vi "Dashboard Main.vi"() -> ()   [LabVIEW 2016]
uses:
  <vilib>/event_ctls.llb/eventvkey.ctl
  <vilib>/Rock Robotics/WPI/Dashboard/WPI_DashboardLogging Global.vi
  <vilib>/Utility/miscctls.llb/LVRowAndColumnTypeDef.ctl
  <vilib>/Rock Robotics/Network Tables/NT Write Boolean.vi
  <vilib>/Rock Robotics/Network Tables/NT Read Numeric Array.vi
panel:
  out "error out":errorcluster
  out "error out 2":errorcluster
  in  "Camera Settings Right":T1={"Frame Rate"=30, "Compression"=30, "Size"=1, "DB Camera Config"=FALSE} {"Frame Rate" scale=1.0..30.0; "Compression" scale=100.0..-1.0; "Size" items=["640x480", "320x240", "160x120"]}
  in  "Camera Name Right":string(combo)="No Camera Selection"
  out "Camera Info":cluster{"Mbps LED":bool, "Mbps":dbl, "fps":dbl} {"fps" format="%#.1g"; "Mbps" format="%#.1g"}
  in  "Camera Settings":T1={"Frame Rate"=30, "Compression"=30, "Size"=1, "DB Camera Config"=FALSE} {"Frame Rate" scale=1.0..30.0; "Compression" scale=100.0..-1.0; "Size" items=["640x480", "320x240", "160x120"]}
  in  "TCP":refnum<k5>
  in  "Rec Mode":enum32{"Stop", "Record", "Playback"}(radio)
  out "Robot IP":string
  out "Image Message":string="Timeout in Camera Communications"
  in  "Dashboard Tab":T2(tab)
  in  "Select Auto":string(combo)="Select Autonomous ..."
  out "NT Connection":bool
  out "MotorChart R":cluster{"Numeric":dbl, "Numeric":dbl}(graph)
  out "MotorChart L":cluster{"Numeric":dbl, "Numeric":dbl}(graph)
  out "MotorSliders R":cluster{"MotorSlide1":dbl, "MotorSlide2":dbl} {"MotorSlide2" scale=-1.0..1.0 scale format="%#_2e"; "MotorSlide1" scale=-1.0..1.0 scale format="%#_2e"}
  out "MotorSliders L":cluster{"MotorSlide1":dbl, "MotorSlide2":dbl} {"MotorSlide2" scale=-1.0..1.0 scale format="%#_2e"; "MotorSlide1" scale=-1.0..1.0 scale format="%#_2e"}
  out "JS1 Z":dbl(slide) scale=-1.0..1.0 scale format="%#_2e"
  out "JS1 Graph":cluster{"X":dbl, "Y":dbl}[](graph)
  out "JS1 Buttons":T3
  out "JS2 Z":dbl(slide) scale=-1.0..1.0 scale format="%#_2e"
  out "JS2 Graph":cluster{"X":dbl, "Y":dbl}[](graph)
  out "JS2 Buttons":T3
  out "Mode":T4(ring)=enum."Auto Disabled"
  out "Gear State":string="Waiting...."
  in  "Mode 2":bool
  out "Camera Image Right":T5(plugin-control)
  in  "DB/String 9":string
  in  "DB/String 8":string
  in  "DB/String 7":string
  in  "DB/String 6":string
  in  "DB/String 5":string
  in  "DB/String 4":string
  in  "DB/String 3":string
  in  "DB/String 2":string
  in  "DB/String 1":string
  in  "DB/String 0":string
  in  "DB/Slider 0":dbl(slide) scale=0.0..5.0
  in  "DB/Slider 1":dbl(slide) scale=0.0..5.0
  in  "DB/Slider 2":dbl(slide) scale=0.0..5.0
  in  "DB/Slider 3":dbl(slide) scale=0.0..5.0
  out "DB/LED 3":bool
  out "DB/LED 2":bool
  out "DB/LED 1":bool
  out "DB/LED 0":bool
  in  "DB/Button 3":bool
  in  "DB/Button 2":bool
  in  "DB/Button 1":bool
  in  "DB/Button 0":bool caption="New Name"
  in  "Test Slider":dbl(slide) scale=0.0..100.0 scale format="%#_3g"
  in  "On/Off":bool caption="Solenoid"
  in  "Test Name":u16(ring) items=["Select the test to run..."]
  in  "Test Tree":string(tree)
  in  "Motor":cluster{"Value":dbl, "Enable":bool} {"Value" scale=-1.0..1.0 scale format="%#_3g"}
  out "Progress":T6 {"Test Progress" scale=0.0..100.0}
  in  "Rev/Fwd":cluster{"Forward":bool, "Reverse":bool}
  in  "Test Ring":u16(ring) items=["Monochrome", "Color"]
  out "Cmd Status":string
  in  "Execute Command":bool
  in  "Command Params":string[][](table)
  in  "Command Selection":i32(listbox)
  in  "CheckList":i32(listbox)
  out "Tree":string(tree)
  in  "Max Speed":dbl=1.0 format="%#_13g"
  in  "Foreward Sensitivity":dbl=1.0 format="%#_13g"
  in  "Turning Sensitivity":dbl=0.4 format="%#_13g"
  in  "High Gear Turning Multiplier":dbl=0.65 format="%#_13g"
  in  "High Gear":bool=TRUE
  in  "Direction Toggle":bool=TRUE
  in  "Autoshift":bool=TRUE
  in  "Save":bool
  in  "Load":bool
  in  "Profile Name":string="Profile1"
  out "Camera Image":T5(plugin-control)
  out "Background":bool
  in  "Camera Name":string(combo)="No Camera Selection"
  # "HW"
  # "HW"
  # "Joysticks"
  # "Drive Motors"
  # "Front"
  # "Right"
  # "Left"
  # "Back"
  # "This tab is a great place for autonomous settings and robot-specific values.\nPlace controls and indicators inside this tab and match name to\nDashboard Variables on robot. You can also delete this comment."
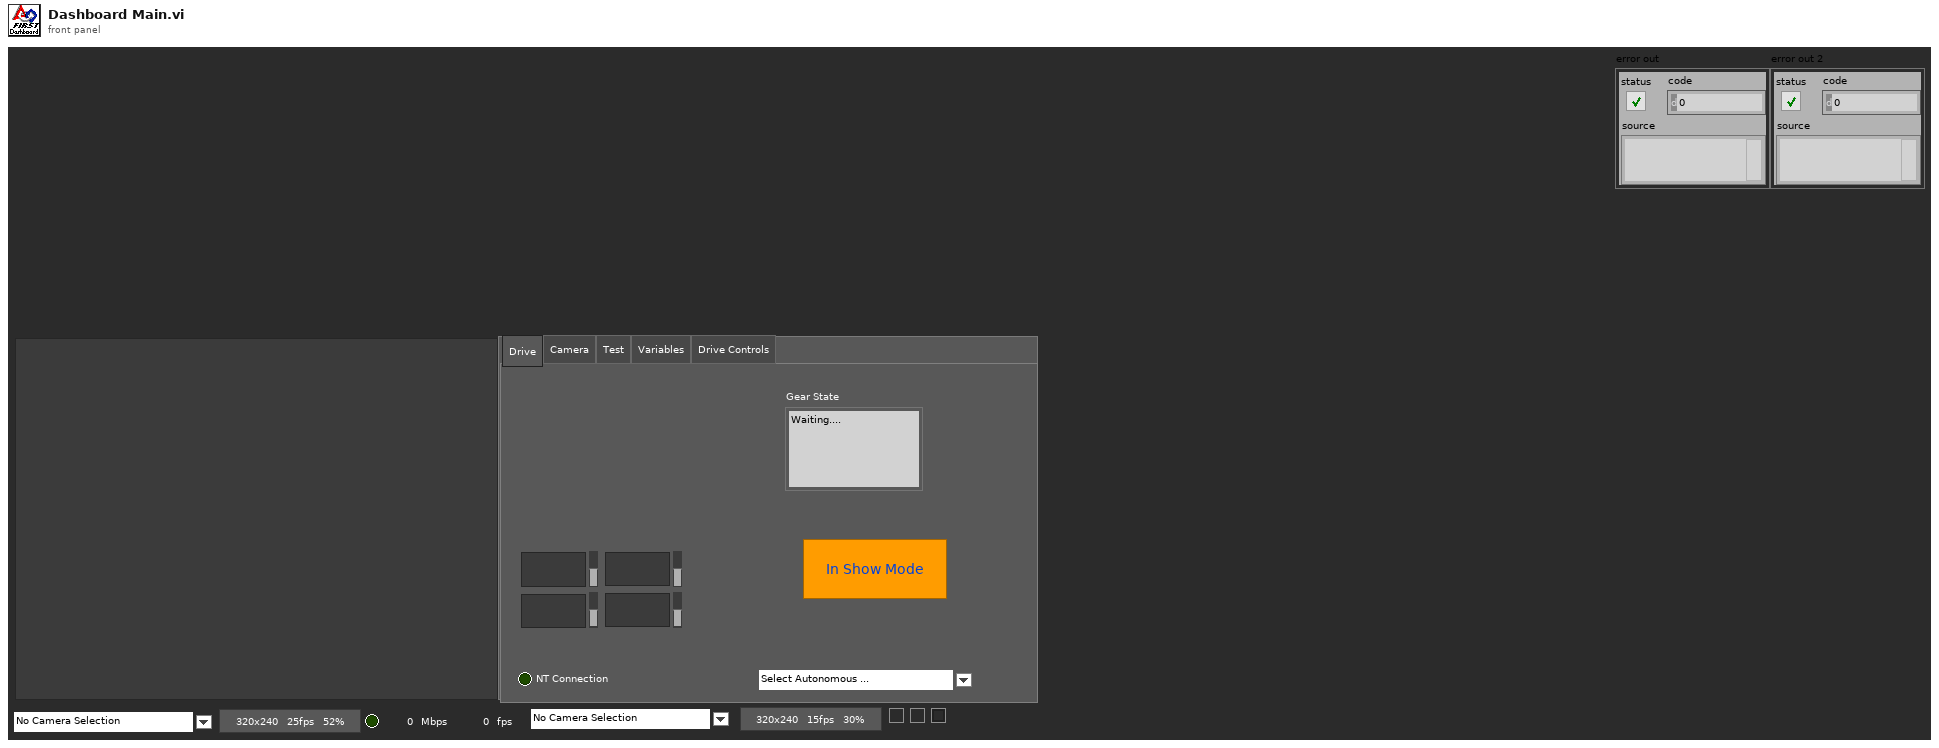
[diagram p1: front panel]
types:
  T1 = cluster{"Frame Rate":i32, "Compression":i32, "Size":u16, "DB Camera Config":bool}
  T2 = enum32{"Drive", "Camera", "Basic", "Custom", "Test", "Commands", "Checklist", "Variables", "Drive Controls"}
  T3 = cluster{bool, bool, bool, bool, bool, bool, bool, bool, bool, bool, bool, bool}
  T4 = enum8{"Tele-Op Disabled", "Tele-Op Enabled", "Auto Disabled", "Auto Enabled", "Test Disabled", "Test Enabled", "Disconnected", "No Code", "E-Stop"}
  T5 = typedef "IMAQ Image.ctl" = refnum<image>
  T6 = cluster{"Test Progress":u8, "Test Progress Text":string}
  T7 = typedef "Image Type" = u32
  T8 = cluster{"IDs":cluster{"RPC field ID":u16, "Unique ID":u16}, "String":string}
  T9 = enum32{"Drive", "Camera", "Basic", "Custom", "Test", "Commands", "Checklist", "Variables"}
  T10 = enum32{"Drive", "Basic", "Custom", "Test", "Checklist", "Variables"}
  T11 = cluster{"Error Strings":string, "Disable Counts":cluster{u16, u16}, "Rail Faults":cluster{u16, u16, u16}, "Robot IP":string, "DB Mode":u8, "Event Info":cluster{"Name":string, "Type":u8, "Number":u16, "Replay":u8}}
  T12 = cluster{"Storage":cluster{"Disk Free":u64, "RAM Block":u32, "RAM free":u32}, "CPU Utilization":cluster{"CPU % ISR":sgl, "CPU % Time Crit":sgl, "CPU % Timed Str":sgl, "CPU % High":sgl, "CPU % Above":sgl, "CPU % Normal":sgl, "CPU % Low":sgl}, "CAN":cluster{"% Bus Utilization":sgl, "Bus Off Cnt":u32, "TX_FIFO Full Cnt":u32, "Receive Error Cnt":u8, "Transmit Error Cnt":u8}, "HID":cluster{"HID Outputs":u32, "Rumble Low":u16, "Rumble High":u16}[]}
  T13 = cluster{"Status bits":cluster{"Test Mode":bool, "Autonomous":bool, "Enabled":bool, "Code Start":bool, "Brownout":bool, "Reserved 2":bool, "Reserved 3":bool, "E-Stop":bool}, "Code Trace":cluster{"Disabled":bool, "TeleOp":bool, "Auto":bool, "Test":bool}, "Controller Type":enum16{"unknown", "cRIO", "roboRio"}, "Code?":enum16{"unknown", "noCode", "code"}, "Battery V":dbl}
  T14 = cluster{"Control Bits":cluster{"TestMode":bool, "Autonomous":bool, "Enabled":bool, "FMS Present":bool, bool, bool, bool, "E-Stop":bool}, "Team Station ":u8, "Countdown":sgl, "Joystick Values":cluster{"Axes":dbl[], "Buttons":bool[], "POVs":i16[]}[]}
  T15 = cluster{"Axes":dbl[], "Buttons":bool[], "POVs":i16[]}[]
  T16 = cluster{"Axes":dbl[], "Buttons":bool[], "POVs":i16[]}
  T17 = cluster{"Buttons[0]":bool, "Buttons[1]":bool, "Buttons[2]":bool, "Buttons[3]":bool, "Buttons[4]":bool, "Buttons[5]":bool, "Buttons[6]":bool, "Buttons[7]":bool, "Buttons[8]":bool, "Buttons[9]":bool, "Buttons[10]":bool, "Buttons[11]":bool}
  T18 = cluster{"Camera Image":refnum<vi>, "Dashboard Tab":refnum<vi>, "Background":refnum<vi>, "Rec Mode":refnum<vi>, "Test Slider":refnum<vi>, "On/Off ":refnum<vi>, "Test Ring":refnum<vi>, "Rev/Fwd":refnum<vi>, "Test Name":refnum<vi>, "Motor":refnum<vi>, "Progress":refnum<vi>, "CheckList":refnum<vi>, "Tree":refnum<vi>, "Test Tree":refnum<vi>, "Command Params":refnum<vi>, "Command Selection":refnum<vi>, "Execute Command":refnum<vi>, "Cmd Status":refnum<vi>, "Camera Settings":refnum<vi>, "Camera Name":refnum<vi>, "Camera Info":refnum<vi>, "Camera Settings Right":refnum<vi>, "Camera Name Right":refnum<vi>, "Camera Image Right":refnum<vi>}
  T19 = cluster{"Operation":enum16{"Update", "Clear"}, "Color Box":u32}[]
  T20 = typedef "eventvkey.ctl" = enum16{"ASCII", "Enter", "Return", "Shift", "Ctrl", "Alt", "Cmd", "Opt", "Caps", "NumLock", "Clear", "Break", "Up", "Down", "Left", "Right", "Insert", "Delete", "Home", "End", "PageUp", "PageDown", "Escape", "Help", "Pause", "ScrollLock", "F1", "F2", "F3", "F4", "F5", "F6", "F7", "F8", "F9", "F10", "F11", "F12", "F13", "F14", "F15", "F16", "F17", "F18", "F19", "F20", "F21", "F22", "F23", "F24", "Play", "VolumeUp", "VolumeDown", "Mute", "Two Byte Char"}
  T21 = cluster{"Image Size":bool, "Image Type":bool, "Pixel Value":bool, "ROI Information":bool, "Zoom Factor":bool}
  T22 = cluster{"Operation":enum16{"Update", "Clear"}, "Color Box":u32}
  T23 = typedef "LVRowAndColumnTypeDef.ctl" = cluster{"Row":i32, "Column":i32}
  T24 = cluster{"Shift":bool, "Ctrl":bool, "Alt":bool, "Cmd":bool, "Opt":bool}
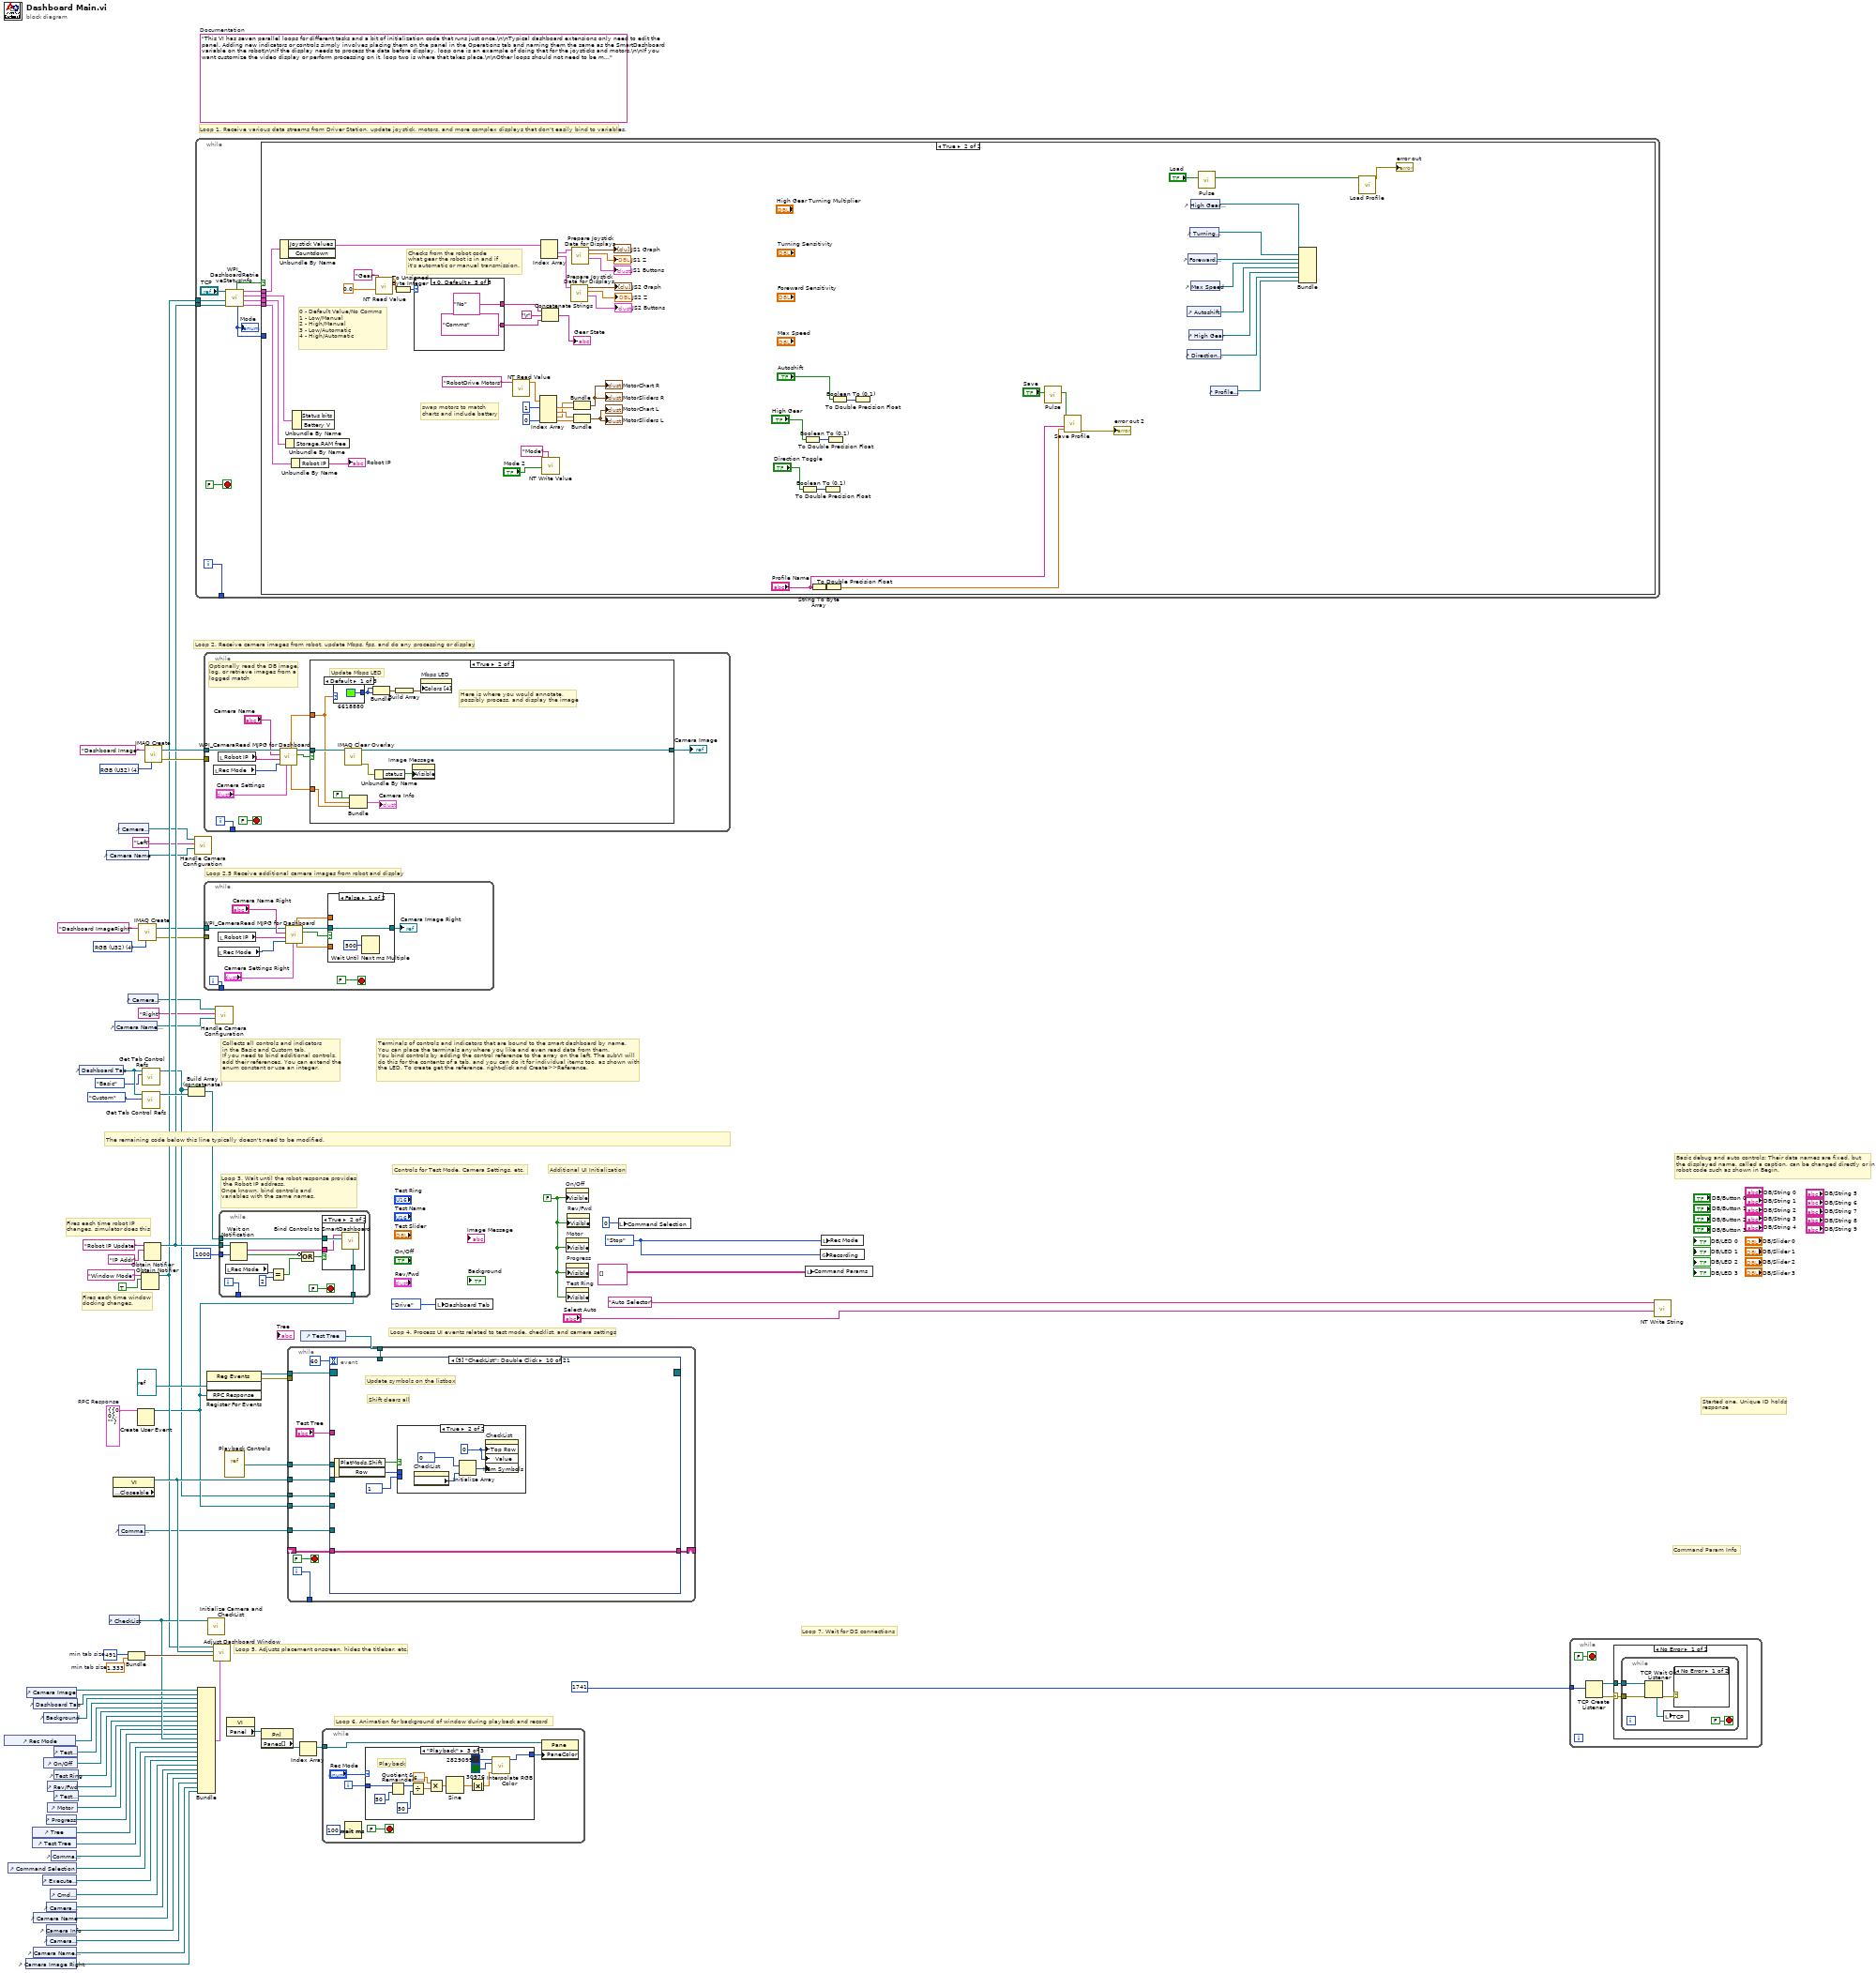
[diagram p0: block diagram]
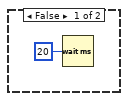
[diagram p3: hidden frame]
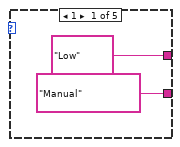
[diagram p4: hidden frame]
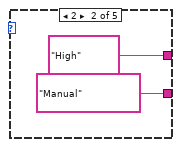
[diagram p5: hidden frame]
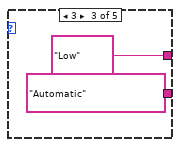
[diagram p6: hidden frame]
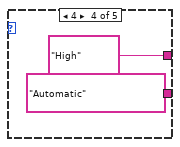
[diagram p7: hidden frame]
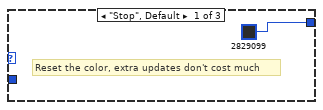
[diagram p8: hidden frame]
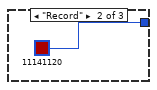
[diagram p9: hidden frame]
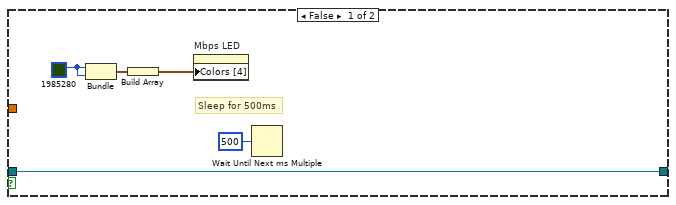
[diagram p11: hidden frame]
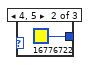
[diagram p12: hidden frame]
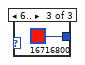
[diagram p13: hidden frame]
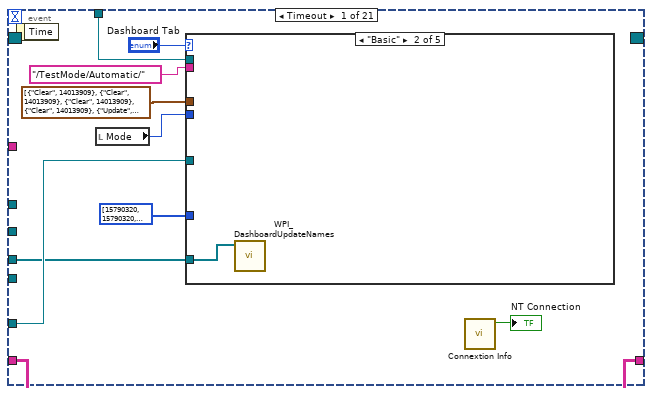
[diagram p14: hidden frame]
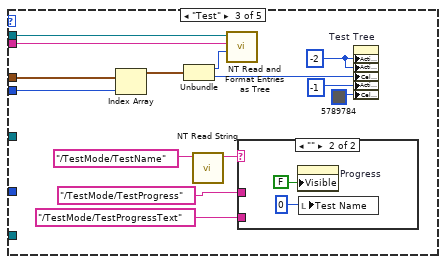
[diagram p16: hidden frame]
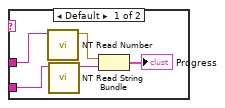
[diagram p17: hidden frame]
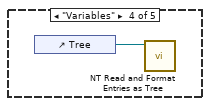
[diagram p18: hidden frame]
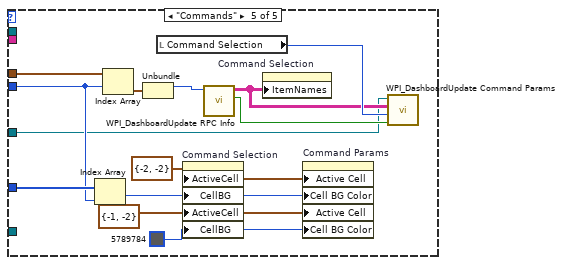
[diagram p19: hidden frame]
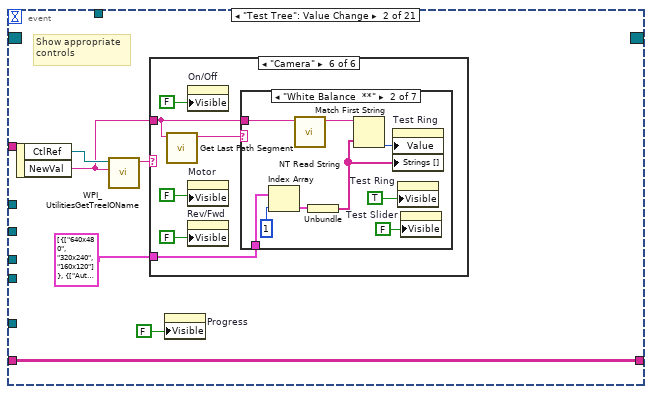
[diagram p20: hidden frame]
diagram:
  w10 = T7 4 items=["Grayscale (U8)", "Grayscale (I16)", "Grayscale (SGL)", "Complex (CSG)", "RGB (U32)", "HSL (U32)", "RGB (U64)"] ("Image Type")
  w26 = T8 {"IDs"={"RPC field ID"=0, "Unique ID"=0}, "String"=""}  # RPC Response
  w51 = 491  # min tab size
  w50 = 1.333  # min tab size
  w58 = enum32{"Stop", "Record", "Playback"}."Stop" ("Rec Mode")
  w33 = FALSE ("Visible")
  (unwired) "This VI has seven parallel loops for different tasks and a bit of initialization code that runs just once.\n\nTypical dashboard extensions only need to edit the panel. Adding new indicators or controls simply involves placing them on the panel in the Operations tab and naming them the same as the SmartDashboard variable on the robot\n\nIf the display needs to process the data before display, loop one is an example of doing that for the joysticks and motors.\n\nIf you want customize the video display or perform processing on it, loop two is where that takes place.\n\nOther loops should not need to be modified. They are pretty standard, and document the task they perform."  # Documentation
  w75 = T7 4 items=["Grayscale (U8)", "Grayscale (I16)", "Grayscale (SGL)", "Complex (CSG)", "RGB (U32)", "HSL (U32)", "RGB (U64)"] ("Image Type")
  # "Loop 2.5 Receive additional camera images from robot and display"
  # "Command Param Info"
  # "Started one, Unique ID holds\nresponse"
  # "Loop 7. Wait for DS connections"
  # "Basic debug and auto controls: Their data names are fixed, but\nthe displayed name, called a caption, can be changed directly or in\nrobot code such as shown in Begin."
  # "Controls for Test Mode, Camera Settings, etc."
  # "Additional UI Initialization"
  # "Loop 6. Animation for background of window during playback and record"
  # "Fires each time robot IP\nchanges, simulator does this"
  # "Fires each time window\ndocking changes."
  # "Collects all controls and indicators\nin the Basic and Custom tab.\nIf you need to bind additional controls,\nadd their references. You can extend the\nenum constant or use an integer."
  # "The remaining code below this line typically doesn't need to be modified."
  # "Loop 4. Process UI events related to test mode, checklist, and camera settings"
  # "Terminals of controls and indicators that are bound to the smart dashboard by name.\nYou can place the terminals anywhere you like and even read data from them.\nYou bind controls by adding the control reference to the array on the left. The subVI will\ndo this for the contents of a tab, and you can do it for individual items too, as shown with\nthe LED. To create get the reference, right-click and Create>>Reference."
  # "Loop 3. Wait until the robot response provides\n the Robot IP address.\nOnce known, bind controls and\nvariables with the same names."
  # "Loop 5. Adjusts placement onscreen, hides the titlebar, etc."
  # "Loop 1. Receive various data streams from Driver Station, update joystick, motors, and more complex displays that don't easily bind to variables."
  # "Loop 2. Receive camera images from robot, update Mbps, fps, and do any processing or display"
  n1 = control-ref of="Rec Mode"() -> (w39:refnum<vi>)
  n2 = control-ref of="Command Selection"() -> (w25:refnum<vi>)
  n3 = control-ref of="Camera Image Right"() -> (w1:refnum<vi>)
  n4 = control-ref of="Camera Image"() -> (w53:refnum<vi>)
  n5 = control-ref of="Tree"() -> (w43:refnum<vi>)
  n6 = control-ref of="Test Tree"() -> (w42:refnum<vi>)
  n7 = control-ref of="Dashboard Tab"() -> (w52:refnum<vi>)
  n8 = control-ref of="Camera Name"() -> (w16:refnum<vi>)
  n9 = control-ref of="Camera Name Right"() -> (w2:refnum<vi>)
  n10 = control-ref of="Execute Command"() -> (w27:refnum<vi>)
  n11 = control-ref of="Background"() -> (w48:refnum<vi>)
  n12 = control-ref of="On/Off"() -> (w37:refnum<vi>)
  n13 = control-ref of="Progress"() -> (w34:refnum<vi>)
  n14 = control-ref of="Camera Settings"() -> (w17:refnum<vi>)
  n15 = control-ref of="Camera Info"() -> (w15:refnum<vi>)
  n16 = control-ref of="Camera Settings Right"() -> (w3:refnum<vi>)
  n17 = control-ref of="Rev/Fwd"() -> (w35:refnum<vi>)
  n18 = control-ref of="Motor"() -> (w40:refnum<vi>)
  n19 = control-ref of="Cmd Status"() -> (w21:refnum<vi>)
  n20 = control-ref of="Command Params"() -> (w28:refnum<vi>)
  n21 = control-ref of="Test Slider"() -> (w38:refnum<vi>)
  n22 = control-ref of="Test Ring"() -> (w36:refnum<vi>)
  n23 = control-ref of="Test Name"() -> (w41:refnum<vi>)
  n24 = control-ref of="Dashboard Tab"() -> (w56:refnum<vi>)
  n25 = control-ref of="Camera Name"() -> (w18:refnum<vi>)
  n26 = control-ref of="CheckList"() -> (w44:refnum<vi>)
  n27 = property class="VI" props=["Front Panel.Closeable"]() -> (reference out=w57:refnum<vi>)  [unwired: 2 in, 2 out]
  n28 = control-ref of="Camera Name Right"() -> (w6:refnum<vi>)
  n29 = control-ref of="Camera Settings"() -> (w19:refnum<vi>)
  n30 = control-ref of="Command Params"() -> (w20:refnum<vi>)
  n31 = control-ref of="Camera Settings Right"() -> (w7:refnum<vi>)
  n32 = Bundle("min tab size"=w51, "min tab size"=w50) -> (w49:cluster{"min tab size":i32, "min tab size":dbl})  [unwired: 1 in]
  n33 = Create User Event(user event datatype=w26) -> (user event=w22:refnum<user-event>)  [unwired: 1 in, 1 out]
  n34 = call "IMAQ Create"("Image Name"="Dashboard ImageRight", "Image Type"=w10) -> ("New Image"=w9:T5, "error out"=w8:errorcluster)  [unwired: 2 in, 1 out]
  n35 = Obtain Notifier(name (unnamed)="Window Mode", notification data type=TRUE) -> (notifier out=w31:refnum<notifier>)  [unwired: 2 in, 2 out]
  n36 = call <vilib>:"Get Tab Control Refs.vi"("Page Index"=T10."Basic" ("Dashboard Tab"), "TabControl in"=w56) -> ("ControlsOnPage"=w14:refnum<vi>[])  [unwired: 9 in]
  n37 = call <vilib>:"Get Tab Control Refs.vi"("Page Index"=T10."Custom" ("Dashboard Tab"), "TabControl in"=w56) -> ("ControlsOnPage"=w55:refnum<vi>[])  [unwired: 9 in]
  n38 = Obtain Notifier(name (unnamed)="Robot IP Update", notification data type="IP Addr" ("name (unnamed)")) -> (notifier out=w32:refnum<notifier>)  [unwired: 2 in, 2 out]
  n39 = call "IMAQ Create"("Image Name"="Dashboard Image", "Image Type"=w75) -> ("New Image"=w73:T5, "error out"=w72:errorcluster)  [unwired: 2 in, 1 out]
  n40 = Build Array (concatenate)(w14, w55) -> (w54:refnum<vi>[])
  n41 = call "Handle Camera Configuration.vi"("CameraNameRef"=w18, "Camera File Name"="Left", "ClusterRef"=w19) -> ()  [unwired: 9 in]
  n42 = while {
    tunnel: [w85] -> _
    tunnel: w32 -> [w79]
    tunnel: w31 -> [w76]
    i -> [w85]
    stop <- FALSE stop-if-true
    n43 = call <vilib>:"WPI_DashboardRetrieveStatusInfo.vi"("Binding Refnum"=w79, "Window Mode Notifier"=w76, "TCP Cnx"="TCP") -> ("Power and Errors"=w80:T11, "Robot Metrics"=w83:T12, "Status Info"=w84:T13, "Control Info"=w81:T14, "Robot Mode"=w78:T4, "Process?"=w82:bool)  [unwired: 3 in]
    "Mode" <- w78
    n44 = case shown="True" w82 {
      tunnel: w84 -> [_ w144]
      tunnel: w83 -> [_ w143]
      tunnel: w81 -> [_ w142]
      tunnel: w80 -> [_ w141]
      tunnel: w78 -> [_ _]
      frame False {
        n45 = Wait (ms)(milliseconds to wait=u32 20) -> ()  [unwired: 1 out]
      }
      frame True {
        # "Checks from the robot code\nwhat gear the robot is in and if\nit's automatic or manual transmission."
        # "0 - Default Value/No Comms\n1 - Low/Manual\n2 - High/Manual\n3 - Low/Automatic\n4 - High/Automatic"
        # "swap motors to match\ncharts and include battery"
        n46 = Unbundle By Name(w142) -> ("Joystick Values"=w132:T15)  [unwired: 1 out]
        n47 = Unbundle By Name(w143) -> ()  [unwired: 1 out]
        n48 = Unbundle By Name(w141) -> ("Robot IP"=→"Robot IP":string)
        n49 = Unbundle By Name(w144) -> ()  [unwired: 2 out]
        n50 = call-poly <vilib>:"NT Read Value.vi"("Default Value"=0.0, "Name"="Gear") -> ("Numeric"=w113:dbl)  [unwired: 8 in, 1 out]
        n51 = To Unsigned Byte Integer(number=w113) -> (unsigned 8bit integer=w114:u8)
        n52 = case shown="0, Default" w114 {
          tunnel: ["Low" "High" "Low" "High" "No"] -> w118
          tunnel: ["Manual" "Manual" "Automatic" "Automatic" "Comms"] -> w116
          frame 1 {
          }
          frame 2 {
          }
          frame 3 {
          }
          frame 4 {
          }
          frame 0, Default {
          }
        }
        n53 = call-poly <vilib>:"NT Read Value.vi"("Name"="RobotDrive Motors") -> ("Numeric Array"=w122:dbl[])  [unwired: 9 in, 1 out]
        n54 = Index Array(array=w122, index #1=1, index #4=0) -> (element #1=w136:dbl, element #2=w137:dbl, element #3=w135:dbl, element #4=w140:dbl)  [unwired: 2 in]
        n55 = Index Array(array=w132) -> (element #1=w131:T16, element #2=w127:T16)  [unwired: 2 in]
        n56 = Concatenate Strings(w118, "\r", w116) -> (→"Gear State":string)
        n57 = call-poly <vilib>:"NT Write Value.vi"("Boolean"="Mode 2", "Name"="Mode") -> ()  [unwired: 9 in, 1 out]
        n58 = call "Prepare Joystick Data for Displays.vi"("Joystick Values"=w127) -> ("Buttons"=→"JS2 Buttons":T17, "Z Axis"=→"JS2 Z":dbl, "Cartesian Data"=→"JS2 Graph":cluster{"X axis":dbl, "X axis":dbl}[])  [unwired: 8 in]
        n59 = call "Prepare Joystick Data for Displays.vi"("Joystick Values"=w131) -> ("Buttons"=→"JS1 Buttons":T17, "Z Axis"=→"JS1 Z":dbl, "Cartesian Data"=→"JS1 Graph":cluster{"X axis":dbl, "X axis":dbl}[])  [unwired: 8 in]
        n60 = Bundle("Numeric"=w135, "Numeric"=w136) -> (→"MotorChart R" →"MotorSliders R":cluster{"Numeric":dbl, "Numeric":dbl})  [unwired: 1 in]
        n61 = Bundle("Numeric"=w137, "Numeric"=w140) -> (→"MotorChart L" →"MotorSliders L":cluster{"Numeric":dbl, "Numeric":dbl})  [unwired: 1 in]
        n62 = Boolean To (0,1)(Boolean="Direction Toggle") -> (0, 1=w103:i16)
        n63 = Boolean To (0,1)(Boolean="High Gear") -> (0, 1=w102:i16)
        n64 = String To Byte Array(string="Profile Name") -> (unsigned byte array=w105:u8[])
        n65 = To Double Precision Float(number=w103) -> ()  [unwired: 1 out]
        n66 = To Double Precision Float(number=w105) -> (double precision float=w106:dbl[])
        n67 = To Double Precision Float(number=w102) -> ()  [unwired: 1 out]
        n68 = Boolean To (0,1)(Boolean="Autoshift") -> (0, 1=w101:i16)
        n69 = To Double Precision Float(number=w101) -> ()  [unwired: 1 out]
        n70 = call "Pulse.vi"("Input"="Save") -> ("Output"=w100:bool)  [unwired: 10 in]
        n71 = call "Save Profile.vi"("Array 2"=w106, "Profile Name"="Profile Name", "Output"=w100) -> ("error out"=→"error out 2":errorcluster)  [unwired: 8 in]
        n72 = control-ref of="Direction Toggle"() -> (w89:refnum<vi>)
        n73 = control-ref of="Autoshift"() -> (w91:refnum<vi>)
        n74 = control-ref of="Foreward Sensitivity"() -> (w93:refnum<vi>)
        n75 = control-ref of="High Gear"() -> (w90:refnum<vi>)
        n76 = control-ref of="Turning Sensitivity"() -> (w94:refnum<vi>)
        n77 = control-ref of="High Gear Turning Multiplier"() -> (w95:refnum<vi>)
        n78 = control-ref of="Max Speed"() -> (w92:refnum<vi>)
        n79 = call "Pulse.vi"("Input"="Load") -> ("Output"=w97:bool)  [unwired: 10 in]
        n80 = control-ref of="Profile Name"() -> (w88:refnum<vi>)
        n81 = Bundle("High Gear Turning Multiplier"=w95, "Turning Sensitivity"=w94, "Foreward Sensitivity"=w93, "Max Speed"=w92, "Autoshift"=w91, "High Gear"=w90, "Direction Toggle"=w89, "Profile Name"=w88) -> ()  [unwired: 1 in, 1 out]
        n82 = call "Load Profile.vi"("Output"=w97) -> ("error out"=→"error out":errorcluster)  [unwired: 14 in]
      }
    }
  }
  n83 = Bundle("Camera Image"=w53, "Dashboard Tab"=w52, "Background"=w48, "Rec Mode"=w39, "Test Slider"=w38, "On/Off"=w37, "Test Ring"=w36, "Rev/Fwd"=w35, "Test Name"=w41, "Motor"=w40, "Progress"=w34, "CheckList"=w44, "Tree"=w43, "Test Tree"=w42, "Command Params"=w28, "Command Selection"=w25, "Execute Command"=w27, "Cmd Status"=w21, "Camera Settings"=w17, "Camera Name"=w16, "Camera Info"=w15, "Camera Settings Right"=w3, "Camera Name Right"=w2, "Camera Image Right"=w1) -> (w45:T18)  [unwired: 1 in]
  n84 = while {
    tunnel: w73 -> [w164]
    tunnel: w72 -> [_]
    tunnel: [w165] -> _
    i -> [w165]
    stop <- FALSE stop-if-true
    # "Optionally read the DB image,\nlog, or retrieve images from a\nlogged match"
    n85 = local read "Rec Mode"() -> (w160:enum32{"Stop", "Record", "Playback"})
    n86 = local read "Robot IP"() -> (w159:string)
    n87 = call <vilib>:"WPI_CameraRead MJPG for Dashboard.vi"("Camera Settings"="Camera Settings", "Rec Mode"=w160, "Robot IP"=w159, "Camera Name"="Camera Name", "Refnum in"=w164) -> ("Active"=w162:bool, "Refnum out"=w163:T5, "FPS"=w161:dbl, "Bandwidth (Mbps)"=w158:dbl)  [unwired: 3 in]
    n88 = case shown="True" w162 {
      tunnel: w163 -> [w167 w178]
      tunnel: w158 -> [_ w175]
      tunnel: w161 -> [_ w176]
      tunnel: [w167 w172] -> w155
      frame False {
        w169 = u32 1985280 ("Color Box")
        # "Sleep for 500ms"
        n89 = Bundle("Color Box"=w169, "Color Box"=w169) -> (w170:cluster{"Color Box":u32, "Color Box":u32})  [unwired: 1 out]
        n90 = Build Array(w170) -> (w168:cluster{"Color Box":u32, "Color Box":u32}[])
        n91 = property on="Mbps LED" class="Bool (strict)"("Colors [4]"=w168) -> ()  [unwired: 2 in, 2 out]
        n92 = Wait Until Next ms Multiple(millisecond multiple=u32 500) -> ()  [unwired: 1 out]
      }
      frame True {
        # "Here is where you would annotate,\npossibly process, and display the image"
        # "Update Mbps LED"
        n93 = case shown="Default" w175 {
          tunnel: [u32 6618880 ("Color Box") u32 16776722 ("Color Box") u32 16716800 ("Color Box")] -> w179
          frame Default {
          }
          frame 4, 5 {
          }
          frame 6.. {
          }
        }
        n94 = call "IMAQ Clear Overlay"("Image"=w178) -> ("error out"=w181:errorcluster, "Image Out"=w172:T5)  [unwired: 2 in, 7 out]
        n95 = Bundle(FALSE, "Bandwidth (Mbps)"=w175, "FPS"=w176) -> (→"Camera Info":cluster{bool, "Bandwidth (Mbps)":dbl, "FPS":dbl})  [unwired: 1 in]
        n96 = Bundle("Color Box"=w179, "Color Box"=w179) -> (w180:cluster{"Color Box":u32, "Color Box":u32})  [unwired: 1 out]
        n97 = Unbundle By Name(w181) -> ("status"=w182:bool)
        n98 = Build Array(w180) -> (w177:cluster{"Color Box":u32, "Color Box":u32}[])
        n99 = property on="Image Message" class="Str"("Visible"=w182) -> ()  [unwired: 2 in, 2 out]
        n100 = property on="Mbps LED" class="Bool (strict)"("Colors [4]"=w177) -> ()  [unwired: 2 in, 2 out]
      }
    }
    "Camera Image" <- w155
  }
  n101 = while {
    tunnel: w9 -> [w196]
    tunnel: w8 -> [_]
    tunnel: [w190] -> _
    i -> [w190]
    stop <- FALSE stop-if-true
    n102 = local read "Rec Mode"() -> (w194:enum32{"Stop", "Record", "Playback"})
    n103 = local read "Robot IP"() -> (w195:string)
    n104 = call <vilib>:"WPI_CameraRead MJPG for Dashboard.vi"("Camera Settings"="Camera Settings Right", "Rec Mode"=w194, "Robot IP"=w195, "Camera Name"="Camera Name Right", "Refnum in"=w196) -> ("Active"=w189:bool, "Refnum out"=w192:T5, "FPS"=w187:dbl, "Bandwidth (Mbps)"=w188:dbl)  [unwired: 3 in]
    n105 = case shown="False" w189 {
      tunnel: w192 -> [w198 w200]
      tunnel: w188 -> [_ _]
      tunnel: w187 -> [_ _]
      tunnel: [w198 w200] -> w186
      frame False {
        n106 = Wait Until Next ms Multiple(millisecond multiple=u32 500) -> ()  [unwired: 1 out]
      }
      frame True {
      }
    }
    "Camera Image Right" <- w186
  }
  n107 = register-events(refnum<vi> refnum, w22) -> (reference out=w62:refnum<event-registration>, error out=w61:errorcluster)  [unwired: 2 in]
  n108 = call "Initialize Camera and CheckList.vi"("ListBox in"=w44) -> ()  [unwired: 11 in]
  n109 = call "Adjust Dashboard Window.vi"("Sizing Refnums"=w45, "Size Constraints"=w49, "VI"=w57, "WIn Mode"=w31) -> ()  [unwired: 8 in]
  n110 = call "Handle Camera Configuration.vi"("CameraNameRef"=w6, "Camera File Name"="Right", "ClusterRef"=w7) -> ()  [unwired: 9 in]
  n111 = while {
    tunnel: w54 -> [w212]
    tunnel: w32 -> [w210]
    tunnel: [w208] -> _
    tunnel: u32 1000 ("milliseconds to wait") -> [w207]
    tunnel: w22 -> [w201]
    i -> [w208]
    stop <- FALSE stop-if-true
    n112 = local read "Rec Mode"() -> (w203:enum32{"Stop", "Record", "Playback"})
    n113 = Wait on Notification(notifier=w210, timeout in ms (-1)=w207) -> (notification=w209:string, timed out?=w205:bool)  [unwired: 2 in, 2 out]
    n114 = Equal?(x=w203, y=u16 2 ("Rec Mode")) -> (x = y?=w204:bool)
    n115 = Compound Arithmetic op=OR(invert w205, w204) -> (w206:bool)
    n116 = case shown="True" w206 {
      tunnel: w212 -> [_ w215]
      tunnel: w209 -> [_ w214]
      tunnel: w201 -> [_ w213]
      frame False {
      }
      frame True {
        n117 = call <vilib>:"Bind Controls to SmartDashboard.vi"("RPC ref"=w213, "Bound Control Refs"=w215, "Server IP Address"=w214) -> ()  [unwired: 9 in]
      }
    }
  }
  n118 = vi-ref "Playback Controls.vi"() -> (w63:refnum<vi>)
  n119 = property class="VI"() -> ("Panel"=w65:refnum<vi>)  [unwired: 2 in, 2 out]
  n120 = property class="Pnl"(reference=w65) -> ("Panes[]"=w66:refnum<vi>[])  [unwired: 1 in, 2 out]
  n121 = Index Array(array=w66) -> (element=w64:refnum<vi>)  [unwired: 1 in]
  n122 = control-ref of="Test Tree"() -> (w67:refnum<vi>)
  n123 = while {
    tunnel: [w225] -> _
    tunnel: w67 -> [w224]
    tunnel: w63 -> [w223]
    tunnel: w62 -> [w222]
    tunnel: w61 -> [_]
    tunnel: w57 -> [w221]
    tunnel: w22 -> [w220]
    tunnel: w20 -> [w219]
    shift-right: [w218] -> _
    shift-left: _ -> [w217]
    tunnel: w14 -> [w216]
    i -> [w225]
    stop <- FALSE stop-if-true
    n124 = event shown="[9] \"CheckList\": Double Click" {
      selector: w222 -> [_ _ _ _ _ _ _ _ _ _ _ _ _ _ _ _ _ _ _ _ _]
      dyn-events: [_ _ _ _ _ _ _ _ _ _ _ _ _ _ _ _ w481 _ _ _ _] -> _
      timeout: u32 60 ("milliseconds to wait") -> [_ _ _ _ _ _ _ _ _ _ _ _ _ _ _ _ _ _ _ _ _]
      tunnel: w224 -> [w237 _ _ _ _ _ _ _ _ _ _ _ _ _ _ _ _ _ _ _ _]
      tunnel: "Test Tree" -> [_ _ _ _ _ _ _ _ _ _ _ w448 w456 w458 w462 w470 _ _ _ _ _]
      tunnel: w223 -> [_ _ _ _ _ _ _ _ _ _ _ _ _ _ _ _ w483 _ w501 _ _]
      tunnel: w221 -> [_ _ _ _ _ _ _ _ _ _ _ _ _ _ _ _ w479 _ _ _ _]
      tunnel: w220 -> [_ _ _ _ _ _ _ _ _ _ _ _ _ _ _ _ w475 _ _ _ _]
      tunnel: w219 -> [w232 _ _ _ _ _ w399 _ _ _ _ _ _ _ _ _ _ _ _ _ _]
      tunnel: [w231 w276 w378 w383 w392 w396 w397 w406 w416 w423 w435 w447 w454 w457 w461 w469 w474 w496 w498 w502 w513] -> w218
      tunnel: w217 -> [w231 w276 w378 w383 w392 w396 w397 _ _ w423 w435 w447 w454 w457 w461 w469 w474 w496 w498 w502 w513]
      tunnel: w216 -> [w229 _ _ _ _ _ _ _ _ _ _ _ _ _ _ _ _ _ _ _ _]
      event Timeout {
        n125 = event-data() -> ()  [unwired: 1 in, 1 out]
        n126 = local read "Mode"() -> (w234:T4)
        n127 = case shown="\"Basic\"" "Dashboard Tab" {
          tunnel: w237 -> [_ _ w253 _ _]
          tunnel: "/TestMode/Automatic/" ("Name Pattern") -> [_ _ w252 _ _]
          tunnel: T19 [{"Operation"=enum."Clear", "Color Box"=14013909}, {"Operation"=enum."Clear", "Color Box"=14013909}, {"Operation"=enum."Clear", "Color Box"=14013909}, {"Operation"=enum."Clear", "Color Box"=14013909}, {"Operation"=enum."Update", "Color Box"=14013909}, {"Operation"=enum."Update", "Color Box"=16777215}, {"Operation"=enum."Clear", "Color Box"=14013909}, {"Operation"=enum."Clear", "Color Box"=14013909}, {"Operation"=enum."Clear", "Color Box"=14013909}] -> [_ _ w245 _ w269]
          tunnel: w234 -> [_ _ w244 _ w268]
          tunnel: u32[] [15790320, 15790320, 15790320, 15790320, 16777215, 16777215, 15790320, 15790320, 15790320] -> [_ _ _ _ w274]
          tunnel: w232 -> [_ _ _ _ w262]
          tunnel: w229 -> [_ w239 _ _ _]
          frame "Custom", Default {
          }
          frame "Basic" {
            n128 = call <vilib>:"WPI_DashboardUpdateNames.vi"("Controls on Tab"=w239) -> ()  [unwired: 11 in]
          }
          frame "Test" {
            w251 = -2 ("Active Item:Row Number")
            n129 = Index Array(array=w245, index=w244) -> (element=w246:T22)
            n130 = Unbundle(w246) -> ("Operation"=w247:enum16{"Update", "Clear"}, "Color Box"=w248:u32)
            n131 = call <vilib>:"NT Read String.vi"("Name"="/TestMode/TestName") -> ("String"=w242:string)  [unwired: 9 in, 1 out]
            n132 = call <vilib>:"NT Read and Format Entries as Tree.vi"("Operation"=w247, "Name Pattern"=w252, "Tree Refnum"=w253) -> ()  [unwired: 7 in, 2 out]
            n133 = case shown="\"\"" w242 {
              tunnel: "/TestMode/TestProgress" ("Name") -> [w255 _]
              tunnel: "/TestMode/TestProgressText" ("Name") -> [w254 _]
              frame Default {
                n134 = call <vilib>:"NT Read Number.vi"("Name"=w255) -> ("Numeric"=w256:dbl)  [unwired: 9 in, 1 out]
                n135 = call <vilib>:"NT Read String.vi"("Name"=w254) -> ("String"=w257:string)  [unwired: 9 in, 1 out]
                n136 = Bundle("Numeric"=w256, "String"=w257) -> (→"Progress":cluster{"Numeric":dbl, "String":string})  [unwired: 1 in]
              }
              frame "" {
                n137 = property on="Progress" class="Clust (strict)"("Visible"=FALSE) -> ()  [unwired: 2 in, 2 out]
                n138 = local write "Test Name"(u16 0) -> ()
              }
            }
            n139 = property on="Test Tree" class="Tree (strict)"("Active Item Row Number"=w251, "ActiveColNum"=w251, "CellBG"=w248, "Active Item Row Number"=-1 ("Active Item:Row Number"), "CellBG"=u32 5789784 ("Color Box")) -> ()  [unwired: 2 in, 2 out]
          }
          frame "Variables" {
            n140 = control-ref of="Tree"() -> (w261:refnum<vi>)
            n141 = call <vilib>:"NT Read and Format Entries as Tree.vi"("Tree Refnum"=w261) -> ()  [unwired: 9 in, 2 out]
          }
          frame "Commands" {
            w270 = u32 5789784 ("Color Box")
            w271 = T23 {"Row"=-1, "Column"=-2} ("Active Cell:Active Cell")
            w273 = T23 {"Row"=-2, "Column"=-2} ("Active Cell:Active Cell")
            n142 = Index Array(array=w274, index=w268) -> (element=w272:u32)
            n143 = Index Array(array=w269, index=w268) -> (element=w267:T22)
            n144 = Unbundle(w267) -> ("Operation"=w266:enum16{"Update", "Clear"})  [unwired: 1 out]
            n145 = local read "Command Selection"() -> (w265:i32)
            n146 = property on="Command Selection" class="MCListbox (strict)"("ActiveCell"=w273, "CellBG"=w272, "ActiveCell"=w271, "CellBG"=w270) -> ()  [unwired: 2 in, 2 out]
            n147 = call <vilib>:"WPI_DashboardUpdate RPC Info.vi"("Operation"=w266) -> ("update"=w264:bool, "commands"=w263:string[][])  [unwired: 9 in]
            n148 = property on="Command Selection" class="MCListbox (strict)"("ItemNames"=w263) -> ()  [unwired: 2 in, 2 out]
            n149 = property on="Command Params" class="Tbl (strict)"("Active Cell"=w273, "Cell BG Color"=w272, "Active Cell"=w271, "Cell BG Color"=w270) -> ()  [unwired: 2 in, 2 out]
            n150 = call <vilib>:"WPI_DashboardUpdate Command Params.vi"("Update"=w264, "NewVal"=w265, "Commands"=w263, "Param Tbl"=w262) -> ()  [unwired: 7 in, 1 out]
          }
        }
        n151 = call <vilib>:"Connextion Info.vi"() -> ("Connected"=→"NT Connection":bool)  [unwired: 10 in, 1 out]
      }
      event "Test Tree": Value Change {
        # "Show appropriate\ncontrols"
        n152 = event-data() -> ("CtlRef"=w279:refnum<vi>, "NewVal"=w277:string)  [unwired: 1 in]
        n153 = call <vilib>:"WPI_UtilitiesGetTreeIOName.vi"("NewVal"=w277, "TreeControl in"=w279) -> ("I/O Name"=w280:string)  [unwired: 9 in]
        n154 = case shown="\"Camera\"" w280 {
          selector: w280 -> [_ w287 _ w309 w318 _]
          tunnel: w277 -> [_ _ w306 w308 _ w325]
          tunnel: cluster{string[]}[] [{["640x480", "320x240", "160x120"]}, {["Auto", "Fixed indoor", "Fixed outdoor 1", "Fixed outdoor 2", "Fixed fluorescent 1", "Fixed fluorescent 2", "Hold current"]}, {["Auto", "Flicker-free 50 Hz", "Flicker-free 60 Hz", "Hold current"]}, {["None", "Prioritize frame rate", "Prioritize image quality"]}, {["Monochrome", "Color"]}] -> [_ _ _ _ _ w324]
          frame Default {
            w282 = FALSE ("Visible")
            w281 = FALSE ("Visible")
            n155 = property on="Motor" class="Clust (strict)"("Visible"=w281) -> ()  [unwired: 2 in, 2 out]
            n156 = property on="Test Ring" class="Ring (strict)"("Visible"=w281) -> ()  [unwired: 2 in, 2 out]
            n157 = property on="Rev/Fwd" class="Clust (strict)"("Visible"=w282) -> ()  [unwired: 2 in, 2 out]
            n158 = property on="On/Off" class="Bool (strict)"("Visible"=w282) -> ()  [unwired: 2 in, 2 out]
            n159 = property on="Test Slider" class="Slide (strict)"("Visible"=w282) -> ()  [unwired: 2 in, 2 out]
          }
          frame "Analog Out", "Motor", "PWM" {
            w288 = FALSE ("Visible")
            n160 = case shown="\"Analog Out\"" w287 {
              tunnel: [1.0 ("Value") -1.0 ("Value") 0.0 ("Value")] -> w286
              tunnel: [255.0 ("Value") 1.0 ("Value") 5.0 ("Value")] -> w285
              tunnel: [128.0 ("Value") 0.0 ("Value") 0.0 ("Value")] -> w284
              tunnel: [64.0 ("Value") 0.5 ("Value") 1.0 ("Value")] -> w283
              frame "PWM" {
              }
              frame "Motor", Default {
              }
              frame "Analog Out" {
              }
            }
            n161 = property on="Motor" class="Clust (strict)"("Visible"=TRUE) -> ()  [unwired: 2 in, 2 out]
            n162 = property on="Value" class="Slide (strict)"("Value"=w284, "Scale.Minimum"=w286, "Scale.Maximum"=w285, "Scale.Increment"=w283) -> ()  [unwired: 2 in, 2 out]
            n163 = property on="On/Off" class="Bool (strict)"("Visible"=w288) -> ()  [unwired: 2 in, 2 out]
            n164 = property on="Test Slider" class="Slide (strict)"("Visible"=w288) -> ()  [unwired: 2 in, 2 out]
            n165 = property on="Test Ring" class="Ring (strict)"("Visible"=w288) -> ()  [unwired: 2 in, 2 out]
            n166 = property on="Rev/Fwd" class="Clust (strict)"("Visible"=w288) -> ()  [unwired: 2 in, 2 out]
          }
          frame "Servo" {
            w304 = FALSE ("Visible")
            n167 = call <vilib>:"NT Read Number.vi"("Name"=w306) -> ("Numeric"=w305:dbl)  [unwired: 9 in, 1 out]
            n168 = property on="Test Slider" class="Slide (strict)"("Visible"=TRUE, "Scale.Maximum"=170.0 ("Scale.Range:Maximum")) -> ()  [unwired: 2 in, 2 out]
            n169 = local write "Test Slider"(w305) -> ()
            n170 = property on="Motor" class="Clust (strict)"("Visible"=w304) -> ()  [unwired: 2 in, 2 out]
            n171 = property on="Rev/Fwd" class="Clust (strict)"("Visible"=w304) -> ()  [unwired: 2 in, 2 out]
            n172 = property on="On/Off" class="Bool (strict)"("Visible"=w304) -> ()  [unwired: 2 in, 2 out]
            n173 = property on="Test Ring" class="Ring (strict)"("Visible"=w304) -> ()  [unwired: 2 in, 2 out]
          }
          frame "Relay", "Solenoid" {
            w307 = FALSE ("Visible")
            n174 = property on="Motor" class="Clust (strict)"("Visible"=w307) -> ()  [unwired: 2 in, 2 out]
            n175 = property on="Test Slider" class="Slide (strict)"("Visible"=w307) -> ()  [unwired: 2 in, 2 out]
            n176 = Search and Replace String(input string=w308, search string="/Value  **", replace string="/Direction") -> (result string=w314:string)  [unwired: 5 in, 3 out]
            n177 = property on="Test Ring" class="Ring (strict)"("Visible"=w307) -> ()  [unwired: 2 in, 2 out]
            n178 = call <vilib>:"NT Read String.vi"("Name"=w314) -> ("String"=w312:string)  [unwired: 9 in, 1 out]
            n179 = Equal?(x="Both directions", y=w312) -> (x = y?=w310:bool)
            n180 = Not(x=w310) -> (.not. x?=w311:bool)
            n181 = property on="Rev/Fwd" class="Clust (strict)"("Visible"=w310) -> ()  [unwired: 2 in, 2 out]
            n182 = property on="On/Off" class="Bool (strict)"("Visible"=w311, "Caption.Text"=w309) -> ()  [unwired: 2 in, 2 out]
          }
          frame "Compressor", "Digital Out" {
            w317 = FALSE ("Visible")
            # "Get direction and finish"
            n183 = property on="Motor" class="Clust (strict)"("Visible"=w317) -> ()  [unwired: 2 in, 2 out]
            n184 = property on="Test Slider" class="Slide (strict)"("Visible"=w317) -> ()  [unwired: 2 in, 2 out]
            n185 = property on="Test Ring" class="Ring (strict)"("Visible"=w317) -> ()  [unwired: 2 in, 2 out]
            n186 = property on="On/Off" class="Bool (strict)"("Visible"=TRUE, "Caption.Text"=w318) -> ()  [unwired: 2 in, 2 out]
            n187 = property on="Rev/Fwd" class="Clust (strict)"("Visible"=FALSE) -> ()  [unwired: 2 in, 2 out]
          }
          frame "Camera" {
            n188 = call <vilib>:"Get Last Path Segment.vi"("String in"=w325) -> ("String out"=w326:string)  [unwired: 10 in]
            n189 = property on="On/Off" class="Bool (strict)"("Visible"=FALSE) -> ()  [unwired: 2 in, 2 out]
            n190 = property on="Motor" class="Clust (strict)"("Visible"=FALSE) -> ()  [unwired: 2 in, 2 out]
            n191 = property on="Rev/Fwd" class="Clust (strict)"("Visible"=FALSE) -> ()  [unwired: 2 in, 2 out]
            n192 = case shown="\"White Balance  **\"" w326 {
              tunnel: w325 -> [w332 w341 w350 w359 w368 _ w374]
              tunnel: w324 -> [w330 w338 w347 w356 w365 _ _]
              frame "Size  **" {
                n193 = Index Array(array=w330) -> (element=w329:cluster{string[]})  [unwired: 1 in]
                n194 = call <vilib>:"NT Read String.vi"("Name"=w332) -> ("String"=w331:string)  [unwired: 9 in, 1 out]
                n195 = Unbundle(w329) -> (w327:string[])
                n196 = Match First String(2:w327, 3:w331) -> (0:w328:i32)  [unwired: 1 out]
                n197 = property on="Test Ring" class="Ring (strict)"("Value"=w328, "Strings []"=w327) -> ()  [unwired: 2 in, 2 out]
                n198 = property on="Test Ring" class="Ring (strict)"("Visible"=TRUE) -> ()  [unwired: 2 in, 2 out]
                n199 = property on="Test Slider" class="Slide (strict)"("Visible"=FALSE) -> ()  [unwired: 2 in, 2 out]
              }
              frame "White Balance  **" {
                n200 = Index Array(array=w338, index=1) -> (element=w339:cluster{string[]})
                n201 = call <vilib>:"NT Read String.vi"("Name"=w341) -> ("String"=w340:string)  [unwired: 9 in, 1 out]
                n202 = Unbundle(w339) -> (w336:string[])
                n203 = Match First String(2:w336, 3:w340) -> (0:w335:i32)  [unwired: 1 out]
                n204 = property on="Test Ring" class="Ring (strict)"("Value"=w335, "Strings []"=w336) -> ()  [unwired: 2 in, 2 out]
                n205 = property on="Test Ring" class="Ring (strict)"("Visible"=TRUE) -> ()  [unwired: 2 in, 2 out]
                n206 = property on="Test Slider" class="Slide (strict)"("Visible"=FALSE) -> ()  [unwired: 2 in, 2 out]
              }
              frame "Exposure  **" {
                n207 = Index Array(array=w347, index=2) -> (element=w348:cluster{string[]})
                n208 = call <vilib>:"NT Read String.vi"("Name"=w350) -> ("String"=w349:string)  [unwired: 9 in, 1 out]
                n209 = Unbundle(w348) -> (w344:string[])
                n210 = Match First String(2:w344, 3:w349) -> (0:w345:i32)  [unwired: 1 out]
                n211 = property on="Test Ring" class="Ring (strict)"("Value"=w345, "Strings []"=w344) -> ()  [unwired: 2 in, 2 out]
                n212 = property on="Test Ring" class="Ring (strict)"("Visible"=TRUE) -> ()  [unwired: 2 in, 2 out]
                n213 = property on="Test Slider" class="Slide (strict)"("Visible"=FALSE) -> ()  [unwired: 2 in, 2 out]
              }
              frame "Exposure Priority  **" {
                n214 = Index Array(array=w356, index=3) -> (element=w357:cluster{string[]})
                n215 = call <vilib>:"NT Read String.vi"("Name"=w359) -> ("String"=w358:string)  [unwired: 9 in, 1 out]
                n216 = Unbundle(w357) -> (w353:string[])
                n217 = Match First String(2:w353, 3:w358) -> (0:w354:i32)  [unwired: 1 out]
                n218 = property on="Test Ring" class="Ring (strict)"("Value"=w354, "Strings []"=w353) -> ()  [unwired: 2 in, 2 out]
                n219 = property on="Test Ring" class="Ring (strict)"("Visible"=TRUE) -> ()  [unwired: 2 in, 2 out]
                n220 = property on="Test Slider" class="Slide (strict)"("Visible"=FALSE) -> ()  [unwired: 2 in, 2 out]
              }
              frame "Color Enable  **" {
                n221 = Index Array(array=w365, index=4) -> (element=w366:cluster{string[]})
                n222 = call <vilib>:"NT Read String.vi"("Name"=w368) -> ("String"=w367:string)  [unwired: 9 in, 1 out]
                n223 = Unbundle(w366) -> (w362:string[])
                n224 = Match First String(2:w362, 3:w367) -> (0:w363:i32)  [unwired: 1 out]
                n225 = property on="Test Ring" class="Ring (strict)"("Value"=w363, "Strings []"=w362) -> ()  [unwired: 2 in, 2 out]
                n226 = property on="Test Ring" class="Ring (strict)"("Visible"=TRUE) -> ()  [unwired: 2 in, 2 out]
                n227 = property on="Test Slider" class="Slide (strict)"("Visible"=FALSE) -> ()  [unwired: 2 in, 2 out]
              }
              frame Default {
                n228 = property on="Test Ring" class="Ring (strict)"("Visible"=FALSE) -> ()  [unwired: 2 in, 2 out]
                n229 = property on="Test Slider" class="Slide (strict)"("Visible"=FALSE) -> ()  [unwired: 2 in, 2 out]
              }
              frame "Brightness  **", "Color Level  **", "Compression  **", "FPS  **", "Sharpness  **" {
                n230 = call <vilib>:"NT Read Number.vi"("Name"=w374) -> ("Numeric"=w373:dbl)  [unwired: 9 in, 1 out]
                n231 = local write "Test Slider"(w373) -> ()
                n232 = property on="Test Slider" class="Slide (strict)"("Visible"=TRUE, "Scale.Maximum"=100.0 ("Scale.Range:Maximum")) -> ()  [unwired: 2 in, 2 out]
                n233 = property on="Test Ring" class="Ring (strict)"("Visible"=FALSE) -> ()  [unwired: 2 in, 2 out]
              }
            }
          }
        }
        n234 = property on="Progress" class="Clust (strict)"("Visible"=FALSE) -> ()  [unwired: 2 in, 2 out]
      }
      event "Test Name": Mouse Enter {
        # "Populate the ring with the list of tests"
        n235 = event-data() -> ()  [unwired: 1 in, 1 out]
        n236 = call <vilib>:"NT Read String Array.vi"("Name"="/TestMode/TestList") -> ("String Array"=w382:string[])  [unwired: 9 in, 1 out]
        n237 = Build Array (concatenate)("Select the test to run...", w382) -> (w381:string[])
        n238 = property on="Test Name" class="Ring (strict)"("Strings []"=w381) -> ()  [unwired: 2 in, 2 out]
      }
      event "Test Name": Value Change {
        w384 = FALSE ("Visible")
        # "Tell the robot the test name to run"
        n239 = event-data() -> ("NewVal"=w388:u16)  [unwired: 1 in]
        n240 = property on="Test Name" class="Ring (strict)"() -> ("Strings []"=w389:string[])  [unwired: 2 in, 2 out]
        n241 = local write "Progress"(T6 {"Test Progress"=0, "Test Progress Text"=""} ("Progress")) -> ()
        n242 = Index Array(array=w389, index=w388) -> (element=w387:string)
        n243 = call <vilib>:"NT Write String.vi"("String"=w387, "Name"="/TestMode/TestName") -> ()  [unwired: 9 in, 1 out]
        n244 = property on="Progress" class="Clust (strict)"("Visible"=TRUE) -> ()  [unwired: 2 in, 2 out]
        n245 = property on="Motor" class="Clust (strict)"("Visible"=w384) -> ()  [unwired: 2 in, 2 out]
        n246 = property on="Test Slider" class="Slide (strict)"("Visible"=w384) -> ()  [unwired: 2 in, 2 out]
        n247 = property on="On/Off" class="Bool (strict)"("Visible"=w384) -> ()  [unwired: 2 in, 2 out]
        n248 = property on="Rev/Fwd" class="Clust (strict)"("Visible"=w384) -> ()  [unwired: 2 in, 2 out]
        n249 = property on="Test Ring" class="Ring (strict)"("Visible"=w384) -> ()  [unwired: 2 in, 2 out]
      }
      event "Select Auto": Mouse Enter {
        # "Populate the combo box with the list of autonomous options"
        n250 = event-data() -> ()  [unwired: 1 in, 1 out]
        n251 = call <vilib>:"NT Read String Array.vi"("Name"="Auto List") -> ("String Array"=w391:string[])  [unwired: 9 in, 1 out]
        n252 = property on="Select Auto" class="CmbBox"("Strings[]"=w391) -> ()  [unwired: 2 in, 2 out]
      }
      event "Select Auto": Value Change {
        # "User modified the Auto Selection. Write to NT variable so robot knows."
        n253 = event-data() -> ("NewVal"=w394:string)  [unwired: 1 in]
        n254 = call <vilib>:"NT Write String.vi"("String"=w394, "Name"="Auto Selector") -> ()  [unwired: 9 in, 1 out]
      }
      event "Command Selection": Value Change {
        # "Get the params and show in table"
        n255 = event-data() -> ("NewVal"=w400:i32)  [unwired: 1 in]
        n256 = property on="Command Selection" class="MCListbox (strict)"() -> ("ItemNames"=w398:string[][])  [unwired: 2 in, 2 out]
        n257 = call <vilib>:"WPI_DashboardUpdate Command Params.vi"("NewVal"=w400, "Commands"=w398, "Param Tbl"=w399) -> ()  [unwired: 8 in, 1 out]
      }
      event "Execute Command": Value Change {
        # "Started one, Unique ID holds\nresponse"
        n258 = event-data() -> ()  [unwired: 1 in, 1 out]
        n259 = property on="Command Selection" class="MCListbox (strict)"() -> ("ItemNames"=w411:string[][])  [unwired: 2 in, 2 out]
        n260 = Index Array(array=w411, index (row)="Command Selection", index (col)=0) -> (element=w409:string)
        n261 = call <vilib>:"Invoke Commands.vi"("Command Params"="Command Params", "Function Name"=w409) -> ("Params"=w405:u8, "Started"=w404:bool)  [unwired: 7 in, 1 out]
        n262 = Array Subset(array="Command Params", length (row)=w405) -> (w406:string[][])  [unwired: 3 in]
        n263 = Select(t="Executing" ("Cmd Status"), s=w404, f="" ("Cmd Status")) -> (s? t:f=→"Cmd Status":string)
      }
      event "Command Selection": Double Click {
        n264 = event-data() -> ("Row"=w419:i32)  [unwired: 1 in]
        n265 = property on="Command Selection" class="MCListbox (strict)"() -> ("ItemNames"=w422:string[][])  [unwired: 2 in, 2 out]
        n266 = local read "Command Params"() -> (w418:string[][])
        n267 = Index Array(array=w422, index (row)=w419, index (col)=0) -> (element=w420:string)
        n268 = call <vilib>:"Invoke Commands.vi"("Command Params"=w418, "Function Name"=w420) -> ("Params"=w417:u8, "Started"=w412:bool)  [unwired: 7 in, 1 out]
        n269 = Array Subset(array=w418, length (row)=w417) -> (w416:string[][])  [unwired: 3 in]
        n270 = Select(t="Executing" ("Cmd Status"), s=w412, f="" ("Cmd Status")) -> (s? t:f=w413:string)
        n271 = local write "Cmd Status"(w413) -> ()
      }
      event "CheckList": Double Click {
        # "Shift clears all"
        # "Update symbols on the listbox"
        n272 = event-data() -> ("PlatMods.Shift"=w424:bool, "Row"=w426:i32)  [unwired: 1 in]
        n273 = case shown="True" w424 {
          tunnel: w426 -> [w430 _]
          tunnel: 1 -> [w429 _]
          frame False {
            n274 = property on="CheckList" class="LstBox (strict)"() -> ("Item Symbols"=w428:i32[])  [unwired: 2 in, 2 out]
            n275 = Replace Array Subset(array=w428, new element=w429, index=w430) -> (w427:i32[])
            n276 = property on="CheckList" class="LstBox (strict)"("Item Symbols"=w427) -> ()  [unwired: 2 in, 2 out]
          }
          frame True {
            w431 = 0 ("Top Row")
            n277 = property on="CheckList" class="LstBox (strict)"() -> ("Number of Rows"=w433:u32)  [unwired: 2 in, 2 out]
            n278 = Initialize Array(0, w433) -> (w432:i32[])
            n279 = property on="CheckList" class="LstBox (strict)"("Top Row"=w431, "Value"=w431, "Item Symbols"=w432) -> ()  [unwired: 2 in, 2 out]
          }
        }
      }
      event "CheckList": Key Down {
        # "Update symbols on the listbox\nLeft and right keys check and uncheck"
        n280 = event-data() -> ("VKey"=w437:T20)  [unwired: 1 in]
        n281 = case shown="\"Left\", \"Right\"" w437 {
          selector: w437 -> [w442 _]
          tunnel: eventvkey."Left" ("VKey") -> [w440 _]
          frame "Left", "Right" {
            n282 = Equal?(x=w440, y=w442) -> (x = y?=w441:bool)
            n283 = Select(t=0, s=w441, f=1) -> (s? t:f=w443:i32)
            n284 = property on="CheckList" class="LstBox (strict)"() -> ("Item Symbols"=w446:i32[])  [unwired: 2 in, 2 out]
            n285 = Replace Array Subset(array=w446, new element=w443, index="CheckList") -> (w445:i32[])
            n286 = property on="CheckList" class="LstBox (strict)"("Item Symbols"=w445) -> ()  [unwired: 2 in, 2 out]
          }
          frame Default {
          }
        }
      }
      event "Motor.Enable": Value Change {
        # "When the test mode otor enable helper is set, update that\ntree row item's value"
        n287 = event-data() -> ("NewVal"=w452:bool)  [unwired: 1 in]
        n288 = Unbundle("Motor") -> ("Value"=w451:dbl)  [unwired: 1 out]
        n289 = Select(t=w451, s=w452, f=0.0) -> (s? t:f=w449:dbl)
        n290 = call <vilib>:"NT Write Number.vi"("Numeric"=w449, "Name"=w448) -> ()  [unwired: 9 in, 1 out]
      }
      event "Test Slider": Value Change {
        # "When the test mode slider helper is set, update that\ntree row item's value"
        n291 = event-data() -> ("NewVal"=w455:dbl)  [unwired: 1 in]
        n292 = call <vilib>:"NT Write Number.vi"("Numeric"=w455, "Name"=w456) -> ()  [unwired: 9 in, 1 out]
      }
      event "On/Off": Value Change {
        # "When the test mode on/off helper value is set, update that\ntree row item's value"
        n293 = event-data() -> ("NewVal"=w460:bool)  [unwired: 1 in]
        n294 = Boolean To (0,1)(Boolean=w460) -> (0, 1=w459:i16)
        n295 = call <vilib>:"NT Write Number.vi"("Numeric"=w459, "Name"=w458) -> ()  [unwired: 9 in, 1 out]
      }
      event "Rev/Fwd": Value Change {
        # "When the test mode helper value for relays is set, update that\ntree row item's value"
        n296 = event-data() -> ("NewVal.Forward"=w468:bool, "NewVal.Reverse"=w467:bool)  [unwired: 1 in]
        n297 = Boolean To (0,1)(Boolean=w468) -> (0, 1=w464:i16)
        n298 = Boolean To (0,1)(Boolean=w467) -> (0, 1=w466:i16)
        n299 = Negate(x=w466) -> (-x=w465:i16)
        n300 = Add(x=w464, y=w465) -> (x+y=w463:i16)
        n301 = call <vilib>:"NT Write Number.vi"("Numeric"=w463, "Name"=w462) -> ()  [unwired: 9 in, 1 out]
      }
      event "Test Ring": Value Change {
        # "When a test mode helper value is selected from the ring,\nset the tree item's variable to the string value"
        n302 = event-data() -> ("NewVal"=w472:u16)  [unwired: 1 in]
        n303 = property on="Test Ring" class="Ring (strict)"() -> ("Strings []"=w473:string[])  [unwired: 2 in, 2 out]
        n304 = Index Array(array=w473, index=w472) -> (element=w471:string)
        n305 = call <vilib>:"NT Write String.vi"("String"=w471, "Name"=w470) -> ()  [unwired: 9 in, 1 out]
      }
      event "Rec Mode": Value Change {
        # "Update globals for recording mode and path to read log from.\nClear when logging and let NetworkTables set path for vision to\nuse."
        n306 = event-data() -> ("NewVal"=w484:enum32{"Stop", "Record", "Playback"})  [unwired: 1 in]
        n307 = global write "WPI_DashboardLogging Global.vi" "Logging Filename"(path "") -> ()
        n308 = global write "WPI_DashboardLogging Global.vi" "Recording"(w484) -> ()
        n309 = case shown="\"Playback\"" w484 {
          tunnel: w483 -> [_ w486 w495]
          tunnel: [_ _ w494] -> w481
          tunnel: [_ _ w493] -> _
          tunnel: w479 -> [_ _ w491]
          tunnel: cluster{i32, i32} {-250, 170} -> [_ _ w490]
          tunnel: [_ _ T21 {"Image Size"=TRUE, "Image Type"=TRUE, "Pixel Value"=TRUE, "ROI Information"=TRUE, "Zoom Factor"=FALSE} ("Image Information Shown:All Elements")] -> w477
          tunnel: [_ _ TRUE ("Zoom Factor")] -> w476
          tunnel: w475 -> [_ _ w487]
          frame Default {
          }
          frame "Stop", "Record" {
            # "Place Window too"
            n310 = invoke class="VI" method="FP.Close"(reference=w486) -> (reference out=w485:refnum<vi>)  [unwired: 2 in, 2 out]
            n311 = invoke class="VI" method="Abort VI"(reference=w485) -> ()  [unwired: 2 in, 3 out]
          }
          frame "Playback" {
            n312 = call "Open Playback Panel.vi"("Offset"=w490, "DB VI Ref"=w491, "Playback in"=w495) -> ("Playback out"=w492:refnum<vi>)  [unwired: 8 in]
            n313 = register-events(w492, w487) -> (reference out=w494:refnum<event-registration>, error out=w493:errorcluster)  [unwired: 2 in]
          }
        }
        n314 = property on="Camera Image" class="ImageControl"("Image Information Shown"=w477, "Image Information Visible"=w476) -> ()  [unwired: 2 in, 2 out]
        n315 = call <vilib>:"WPI_DashboardNT Log FieldName Cache.vi"("Operation"=enum16{"Lookup/Add", "Index", "Clear"}."Clear") -> ()  [unwired: 8 in, 3 out]
      }
      event Panel Close {
        w497 = enum32{"Stop", "Record", "Playback"}."Stop" ("Rec Mode")
        # "Playback window has been closed, abort"
        n316 = event-data() -> ()  [unwired: 1 in, 4 out]
        n317 = local write "Rec Mode"(w497) -> ()
        n318 = global write "WPI_DashboardLogging Global.vi" "Recording"(w497) -> ()
      }
      event Panel Close {
        # "Abort playback window and ourself"
        n319 = event-data() -> ()  [unwired: 1 in, 4 out]
        n320 = invoke class="VI" method="FP.Close"(reference=w501) -> (reference out=w500:refnum<vi>)  [unwired: 2 in, 2 out]
        n321 = invoke class="VI" method="Abort VI"(reference=w500) -> (error out=w499:errorcluster)  [unwired: 2 in, 2 out]
        n322 = invoke class="VI" method="Abort VI"(error in=w499) -> ()  [unwired: 2 in, 3 out]
      }
      event User Event {
        n323 = event-data() -> ("IDs"=w508:cluster{"RPC field ID":u16, "Unique ID":u16}, "String"=w507:string)  [unwired: 1 in]
        n324 = Bundle("IDs"=w508, "String"=w507) -> (w506:T8)  [unwired: 1 in]
        n325 = call <vilib>:"Retrieve RPC Response.vi"("RPC Response"=w506) -> ("Output"=w504:string[][])  [unwired: 10 in]
        n326 = Build Array (concatenate)(w502, w504) -> (w503:string[][])
        n327 = local write "Command Params"(w503) -> ()
        n328 = local write "Cmd Status"("" ("Cmd Status")) -> ()
      }
      event "Tree": Double Click {
        n329 = event-data() -> ("PlatMods"=w512:T24, "Tag"=w511:string)  [unwired: 1 in]
        n330 = Unbundle(w512) -> ("Shift"=w510:bool)  [unwired: 4 out]
        n331 = Not(x=w510) -> (.not. x?=w509:bool)
        n332 = call <vilib>:"NT Update Persistence.vi"("Persistence"=w509, "Name"=w511) -> ()  [unwired: 9 in, 1 out]
      }
    }
  }
  n333 = while {
    tunnel: w64 -> [w515]
    i -> [w518]
    stop <- FALSE stop-if-true
    n334 = Wait (ms)(milliseconds to wait=u32 100) -> ()  [unwired: 1 out]
    n335 = case shown="\"Playback\"" "Rec Mode" {
      tunnel: w518 -> [_ _ w533]
      tunnel: [u32 2829099 ("Base Color") u32 11141120 ("Target Color") w522] -> w514
      frame "Stop", Default {
        # "Reset the color, extra updates don't cost much"
      }
      frame "Record" {
      }
      frame "Playback" {
        # "Playback"
        n336 = Quotient & Remainder(x=w533, y=u32 50 ("milliseconds to wait")) -> (x-y*floor(x/y)=w529:u32)  [unwired: 1 out]
        n337 = Divide(x=w529, y=u32 50 ("milliseconds to wait")) -> (x/y=w526:dbl)
        n338 = Multiply(x=6.283185307179586, y=w526) -> (x*y=w531:dbl)
        n339 = Sine(x=w531) -> (sin(x)=w530:dbl)
        n340 = Absolute Value(x=w530) -> (abs(x)=w523:dbl)
        n341 = call "Interpolate RGB Color.vi"("Proportion"=w523, "Target Color"=u32 30976, "Base Color"=u32 2829099) -> ("Result Color"=w522:u32)  [unwired: 8 in]
      }
    }
    n342 = property class="Pane"(reference=w515, "PaneColor"=w514) -> ()  [unwired: 1 in, 2 out]
  }
  n343 = local write "Dashboard Tab"(T9."Drive" ("Dashboard Tab")) -> ()
  n344 = property on="On/Off" class="Bool (strict)"("Visible"=w33) -> ()  [unwired: 2 in, 2 out]
  n345 = property on="Motor" class="Clust (strict)"("Visible"=w33) -> ()  [unwired: 2 in, 2 out]
  n346 = property on="Progress" class="Clust (strict)"("Visible"=w33) -> ()  [unwired: 2 in, 2 out]
  n347 = property on="Test Ring" class="Ring (strict)"("Visible"=w33) -> ()  [unwired: 2 in, 2 out]
  n348 = property on="Rev/Fwd" class="Clust (strict)"("Visible"=w33) -> ()  [unwired: 2 in, 2 out]
  n349 = local write "Command Selection"(u16 0 ("milliseconds to wait")) -> ()
  n350 = local write "Command Params"(string[][] [] ("Command Params")) -> ()
  n351 = global write "WPI_DashboardLogging Global.vi" "Recording"(w58) -> ()
  n352 = local write "Rec Mode"(w58) -> ()
  n353 = while {
    tunnel: u16 1741 ("timeout ms (25000)") -> [w535]
    stop <- FALSE stop-if-true
    n354 = TCP Create Listener(10:w535) -> (0:w534:errorcluster, 3:w536:refnum<k5>)  [unwired: 4 in, 1 out]
    n355 = case shown="No Error" w534 {
      selector: w534 -> [w538 _]
      tunnel: w536 -> [w539 _]
      frame No Error {
        n356 = while {
          tunnel: w539 -> [w542]
          tunnel: w538 -> [w541]
          stop <- FALSE stop-if-true
          n357 = TCP Wait On Listener(8:w541, 11:w542) -> (0:w543:errorcluster, 4:w544:refnum<k5>)  [unwired: 2 in, 3 out]
          n358 = local write "TCP"(w544) -> ()
          n359 = case shown="No Error" w543 {
            frame No Error {
            }
            frame Error {
              n360 = Wait (ms)(milliseconds to wait=u32 1000) -> ()  [unwired: 1 out]
            }
          }
        }
      }
      frame Error {
        n361 = Wait (ms)(milliseconds to wait=u32 1000) -> ()  [unwired: 1 out]
      }
    }
  }
  n362 = call <vilib>:"NT Write String.vi"("String"="Select Auto", "Name"="Auto Selector") -> ()  [unwired: 9 in, 1 out]
